vi "Simulation_Engine.vi"(0 "Path in":refnum<vi>, 1 "c_s2 [ppmv]":dbl=1.0, 2 "l2 [m]":dbl=1000.0, 3 "l_s [m]":dbl=0.1, 4 "c_s [ppmv]":dbl=1.0, 5 "c [ppmv]":dbl=1.7, 6 "l [m]":dbl=1000.0, 8 "c2 [ppmv]":dbl=7750.0, 9 "Array in":dbl[](array[numeric]), 10 "reference in":refnum<vi>, 11 "R":dbl, 12 "l_S2 [m]":dbl=1.0, 13 "K":dbl, 15 "Boolean":bool, 17 "f_LP1":dbl=1000.0, 19 "f_LP2":dbl=1000.0) -> (7 "I_OUT":cluster{dbl[], dbl[]}(graph), 14 "XY Graph":cluster{dbl[], dbl[]}[](graph), 16 "Widmo drugiej pochodnej":cluster{"f0":dbl, "df":dbl, "magnitude":dbl[]}(graph), 18 "Widmo pierwszej pochodnej":cluster{"f0":dbl, "df":dbl, "magnitude":dbl[]}(graph), 20 "Pierwsza pochodna":cluster{dbl[], dbl[]}(graph), 21 "Druga pochodna":cluster{dbl[], dbl[]}(graph), 23 "1fm":cluster{dbl[], dbl[]}(graph), 24 "2f bg":cluster{dbl[], dbl[]}(graph), 27 "2f/1f":cluster{dbl[], dbl[]}(graph))   [LabVIEW 2019]
uses:
  <vilib>/Analysis/3filter.llb/Filter Passband Type.ctl
  <vilib>/Utility/file.llb/Read Delimited Spreadsheet (DBL).vi
  <vilib>/Analysis/3filter.llb/Butterworth Filter (DBL).vi
  <vilib>/Analysis/baseanly.llb/IIR Cascade Filter (DBL).vi
  <vilib>/express/express analysis/Spectral/Block/exnSpectralBlock spectral measurements power poly.vi
  <vilib>/express/express analysis/Spectral/Block/exnSpectralBlock spectral measurements power WFM.vi
  <vilib>/express/express analysis/Spectral/XNode/ExpressSpectralMeasurementsBlockNode.xnode
  <vilib>/gmath/NI_Gmath.lvlib
  <vilib>/Analysis/NI_AALPro.lvlib
  <vilib>/Analysis/NI_AALBase.lvlib
panel:
  out "2f me":cluster{dbl[], dbl[]}(graph)
  out "1f bg":cluster{dbl[], dbl[]}(graph)
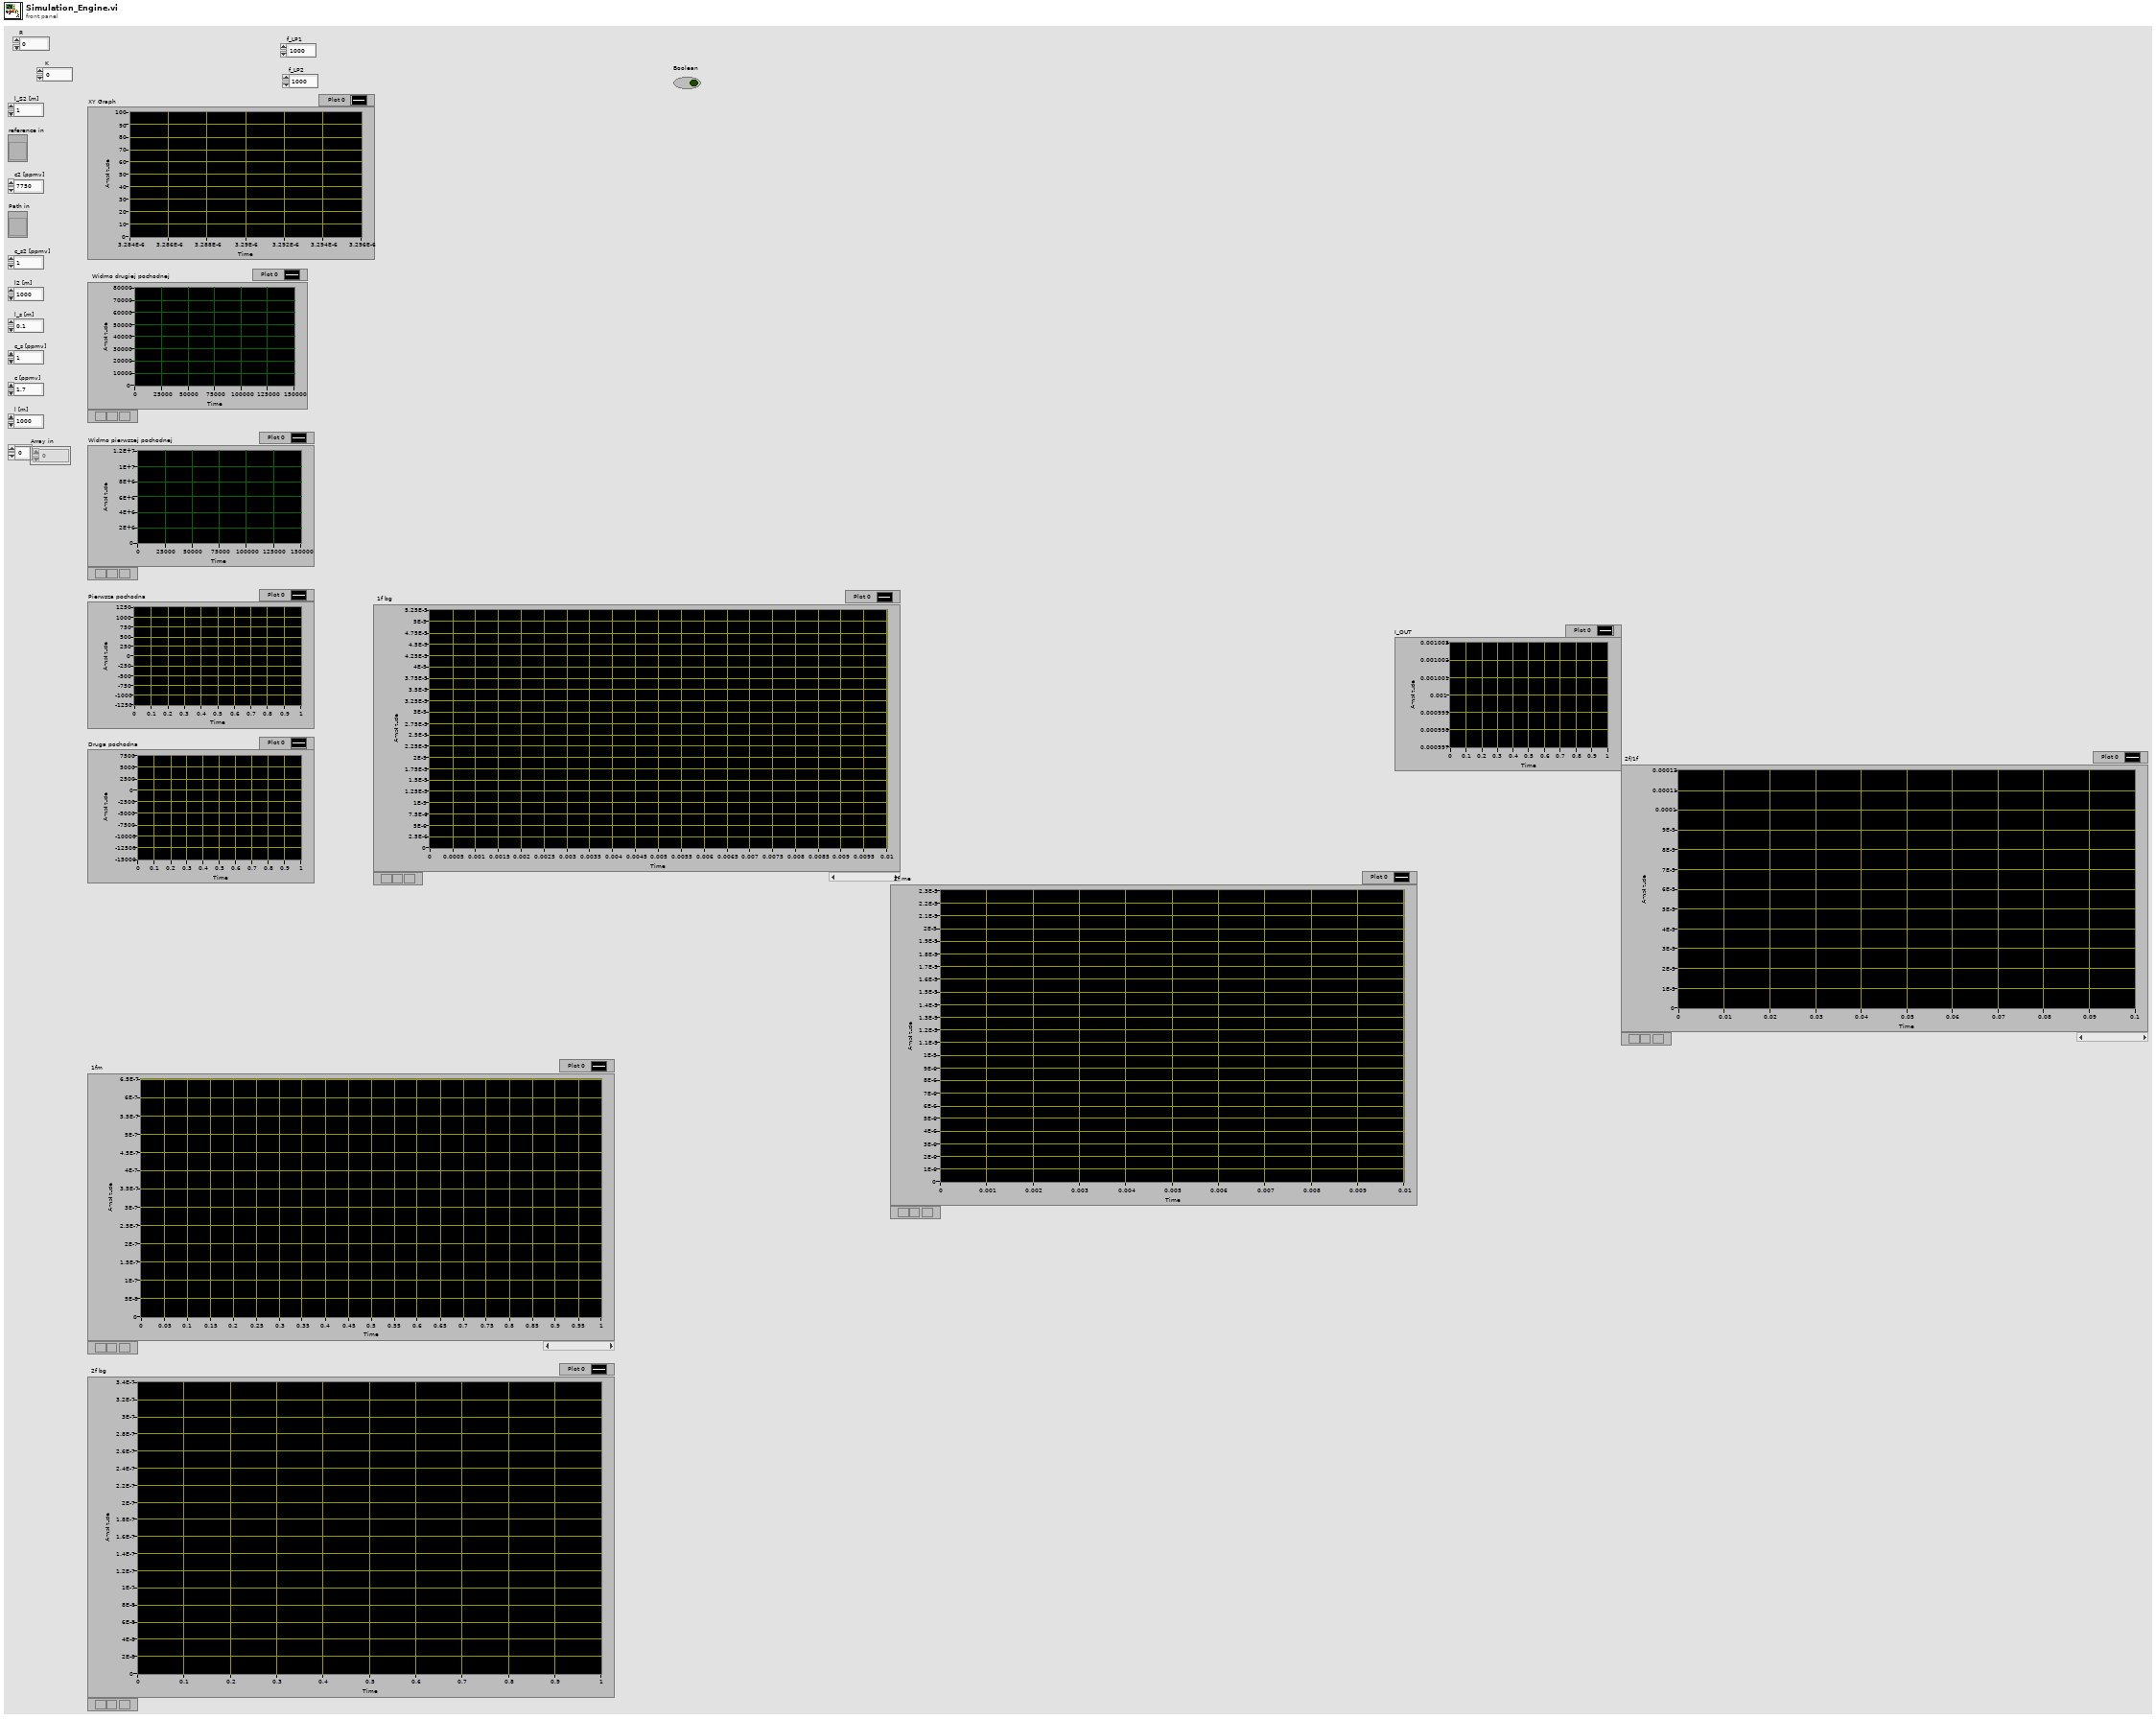
[diagram p1: front panel]
types:
  T1 = typedef "NI_AALBase.lvlib/Filter Passband Type.ctl" = enum32{"Lowpass", "Highpass", "Bandpass", "Bandstop"}
  T2 = cluster{"filter structure":enum32{"IIR 2nd Order", "IIR 4th Order"}, "Reverse Coefficients":dbl[], "Forward Coefficients":dbl[]}
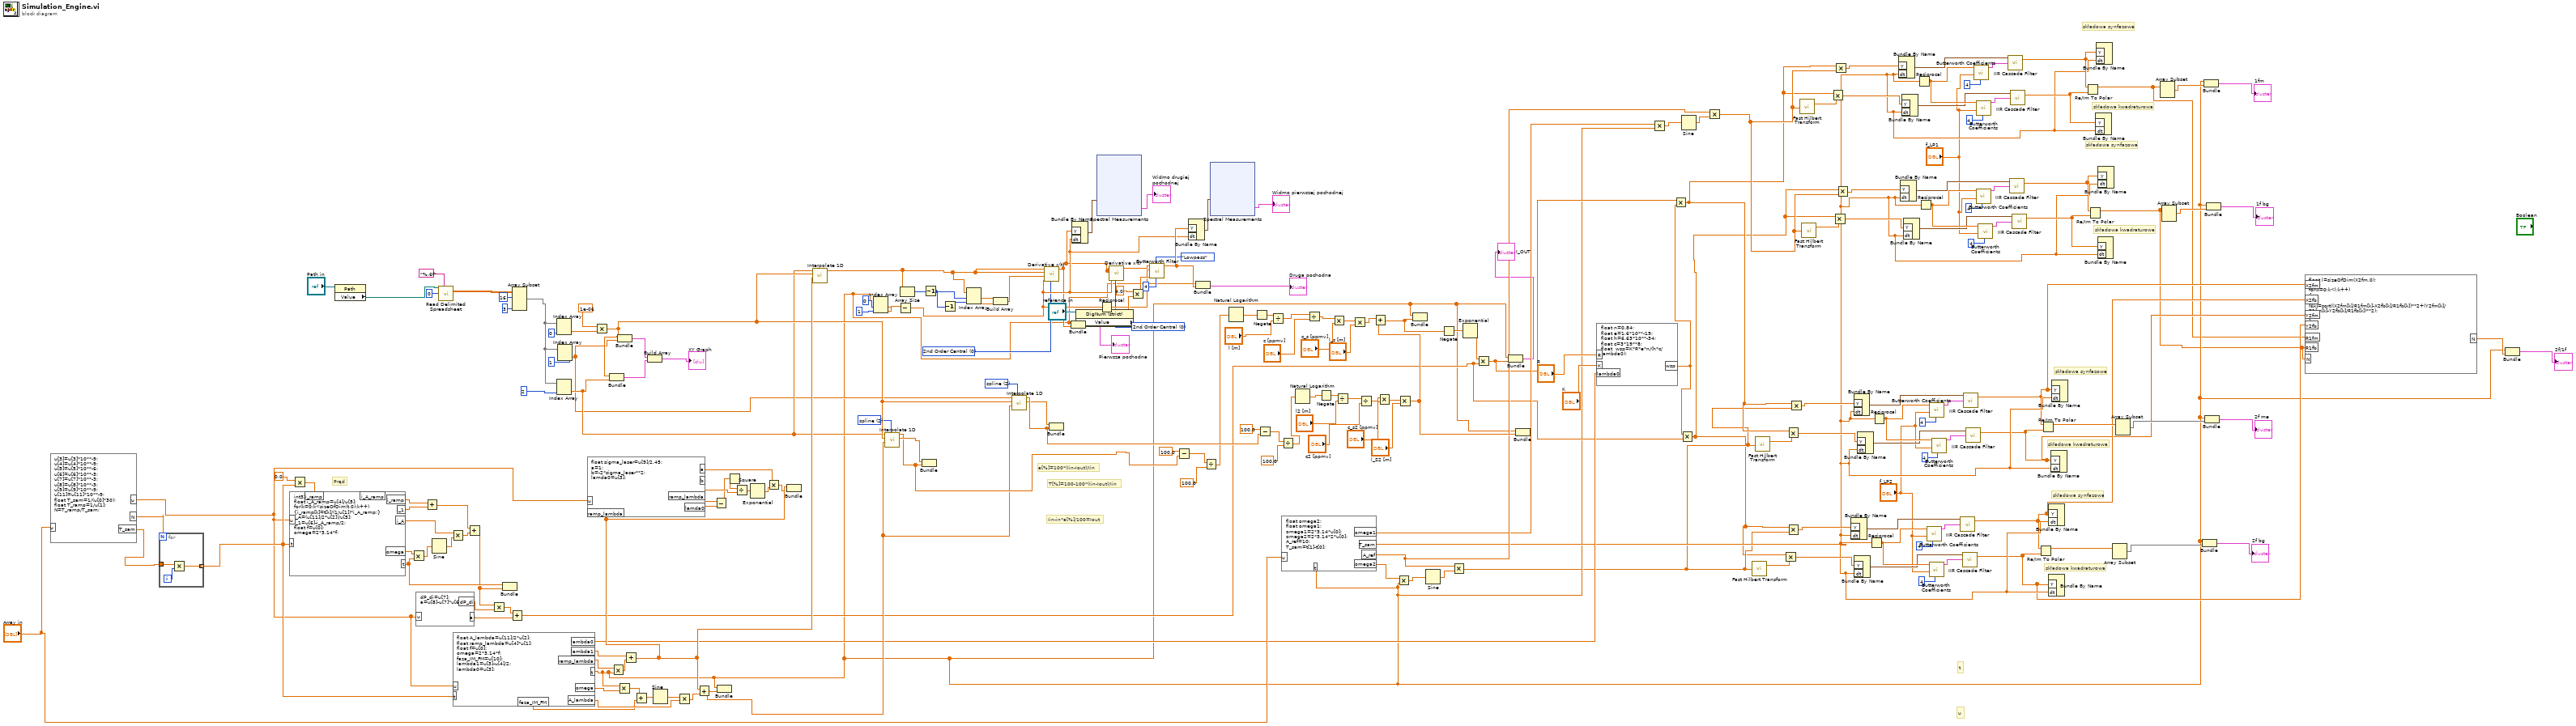
[diagram p0: block diagram]
diagram:
  w179 = u16 0 items=["2nd Order Central", "4th Order Central", "Forward", "Backward"] ("method")
  w170 = u16 0 items=["2nd Order Central", "4th Order Central", "Forward", "Backward"] ("method")
  w109 = 2 items=["nearest", "linear", "spline", "cubic Hermite", "Lagrange"] ("method")
  w106 = 2 items=["nearest", "linear", "spline", "cubic Hermite", "Lagrange"] ("method")
  # "składowa synfazowa"
  # "składowa synfazowa"
  # "składowa synfazowa"
  # "składowa kwadraturowa"
  # "składowa kwadraturowa"
  # "składowa kwadraturowa"
  # "składowa synfazowa"
  # "składowa kwadraturowa"
  # "u"
  # "t"
  # "T[%]=100-100*(Iin-Iout)/Iin"
  # "Iin-in*a[%]/100=Iout"
  # "a[%]=100*(Iin-Iout)/Iin"
  # "Natężenie"
  # "Prąd"
  n1 = formula code="u[3]=u[3]*10**-9;\nu[4]=u[4]*10**-9;\nu[5]=u[5]*10**-6;\nu[6]=u[6]*10**-3;\nu[7]=u[7]*10**-3;\nu[8]=u[8]*10**-3;\nu[9]=u[9]*10**-9;\nu[11]=u[11]*10**-9;\nfloat T_sam=1/(u[0]*30);\nfloat T_ramp=1/u[1];\nN=T_ramp/T_sam;"("u"="Array in") -> ("N"=w87:dbl, "T_sam"=w88:dbl, "u"=w89:dbl[])
  n2 = for {
    N: w87 -> [_]
    tunnel: w88 -> [w214]
    tunnel: [w212] -> w90 mode=indexing
    i -> [w213]
    n3 = Multiply(x=w214, y=w213) -> (x*y=w212:dbl)
  }
  n4 = Multiply(x=0.0, y=w90) -> (x*y=w56:dbl[])
  n5 = formula code="int32 k=0;\nfloat i_A_ramp=u[4]/u[5];\nfor(k=0;k<sizeOfDim(t,0);k++)\n{i_ramp[k]=t[k]/(1/u[1])*i_A_ramp;}\ni_A=(u[11]/2*u[2])/u[5];\ni_1=u[6]-i_A_ramp/2;\nfloat f=u[0];\nomega=2*3.14*f;"("u"=w89, "t"=w90, "i_ramp"=w56) -> ("i_A"=w57:dbl, "i_1"=w91:dbl, "i_ramp"=w59:dbl[], "omega"=w61:dbl, "t"=w190:dbl[])  [unwired: 1 out]
  n6 = property class="Path"(reference="Path in") -> ("Value"=w105:path)  [unwired: 1 in, 2 out]
  n7 = Multiply(x=w61, y=w190) -> (x*y=w62:dbl[])
  n8 = formula code="dP_di=u[7];\na=u[8]-u[7]*u[6];"("u"=w89) -> ("dP_di"=w65:dbl, "a"=w66:dbl)
  n9 = Add(x=w59, y=w91) -> (x+y=w60:dbl[])
  n10 = Sine(x=w62) -> (sin(x)=w63:dbl[])
  n11 = call-poly <vilib>:"Read Delimited Spreadsheet.vi"("file path (dialog if empty)"=w105, "format (%.3f)"="%.6f", "start of read offset (chars.:0)"=0) -> ("all rows"=w95:dbl[][])  [unwired: 7 in, 5 out]
  n12 = Multiply(x=w57, y=w63) -> (x*y=w58:dbl[])
  n13 = formula code="float A_lambda=u[11]/2*u[2];\nfloat ramp_lambda=u[4]*u[1];\nfloat f=u[0];\nomega=2*3.14*f;\nfaza_IM_FM=u[10];\nlambda1=u[3]-u[4]/2;\nlambda0=u[3];"("u"=w89, "t"=w90) -> ("ramp_lambda"=w74:dbl, "t"=w8:dbl[], "omega"=w68:dbl, "faza_IM_FM"=w70:dbl, "A_lambda"=w73:dbl, "lambda1"=w75:dbl, "lambda0"=w25:dbl)
  n14 = Add(x=w60, y=w58) -> (x+y=w64:dbl[])
  n15 = Multiply(x=w64, y=w65) -> (x*y=w67:dbl[])
  n16 = Bundle("t"=w190, w64) -> ()  [unwired: 1 in, 1 out]
  n17 = Add(x=w67, y=w66) -> (x+y=w21:dbl[])
  n18 = Array Subset(array=w95, index (row)=16 ("index"), length (col)=3 ("length")) -> (w94:dbl[][])  [unwired: 2 in]
  n19 = Index Array(array=w94, index (col)=2 ("disabled index (col)")) -> (element=w162:dbl[])  [unwired: 1 in]
  n20 = Index Array(array=w94, index (col)=0 ("disabled index (col)")) -> (element=w107:dbl[])  [unwired: 1 in]
  n21 = Index Array(array=w94, index (col)=1 ("disabled index (col)")) -> (element=w110:dbl[])  [unwired: 1 in]
  n22 = Multiply(x=1e-06, y=w107) -> (x*y=w163:dbl[])
  n23 = Bundle(w163, w162) -> (w93:cluster{dbl[], dbl[]})  [unwired: 1 in]
  n24 = Multiply(x=w74, y=w8) -> (x*y=w85:dbl[])
  n25 = Bundle(w163, w110) -> (w96:cluster{dbl[], dbl[]})  [unwired: 1 in]
  n26 = Multiply(x=w8, y=w68) -> (x*y=w69:dbl[])
  n27 = Add(x=w75, y=w85) -> (x+y=w169:dbl[])
  n28 = formula code="float sigma_laser=u[9]/2.45;\na=1;\nb=-2*sigma_laser**2;\nlamda0=u[3];"("u"=w89, "ramp_lambda"=w169) -> ("b"=w83:dbl, "a"=w78:dbl, "ramp_lambda"=w79:dbl[], "lamda0"=w80:dbl)
  n29 = Add(x=w69, y=w70) -> (x+y=w71:dbl[])
  n30 = Build Array(w96, w93) -> (→"XY Graph":cluster{dbl[], dbl[]}[])
  n31 = Sine(x=w71) -> (sin(x)=w72:dbl[])
  n32 = Multiply(x=w72, y=w73) -> (x*y=w76:dbl[])
  n33 = Add(x=w169, y=w76) -> (x+y=w111:dbl[])
  n34 = Subtract(x=w79, y=w80) -> (x-y=w81:dbl[])
  n35 = Bundle("t"=w8, w111) -> ()  [unwired: 1 in, 1 out]
  n36 = Square(x=w81) -> (x^2=w82:dbl[])
  n37 = Divide(x=w82, y=w83) -> (x/y=w84:dbl[])
  n38 = Exponential(1:w84) -> (0:w77:dbl[])
  n39 = Multiply(x=w78, y=w77) -> (x*y=w86:dbl[])
  n40 = Bundle(w169, w86) -> ()  [unwired: 1 in, 1 out]
  n41 = call <vilib>:"Interpolate 1D.vi"("xi"=w169, "X"=w163, "Y"=w162) -> ("yi"=w171:dbl[])  [unwired: 6 in, 2 out]
  n42 = Index Array(array=w8, index #1=0 ("index"), index #2=1 ("index")) -> (element #1=w164:dbl, element #2=w165:dbl)
  n43 = call <vilib>:"Interpolate 1D.vi"("method"=w106, "xi"=w111, "X"=w163, "Y"=w162) -> ("xi used"=w161:dbl[], "yi"=w160:dbl[])  [unwired: 5 in, 1 out]
  n44 = Subtract(x=w165, y=w164) -> (x-y=w191:dbl)
  n45 = Array Size(array=w171) -> (size(s)=w176:i32)
  n46 = Bundle("xi used"=w161, "yi"=w160) -> ()  [unwired: 1 in, 1 out]
  n47 = Decrement(x=w176) -> (x-1=w177:i32)
  n48 = Decrement(x=w177) -> (x-1=w172:i32)
  n49 = Index Array(array=w171, index #1=w177, index #2=w172) -> (element #1=w173:dbl, element #2=w174:dbl)
  n50 = Build Array(w173, w174) -> (w175:dbl[])
  n51 = call <vilib>:"Interpolate 1D.vi"("method"=w109, "xi"=w111, "X"=w163, "Y"=w110) -> ("xi used"=w108:dbl[], "yi"=w140:dbl[])  [unwired: 5 in, 1 out]
  n52 = call <vilib>:"Derivative x(t).vi"("method"=w170, "dt"=w191, "Final Condition"=w175, "Initial Condition"=w171, "X"=w171) -> ("dX/dt"=w186:dbl[])  [unwired: 5 in, 1 out]
  n53 = Bundle("xi used"=w108, "yi"=w140) -> ()  [unwired: 1 in, 1 out]
  n54 = Bundle("t"=w8, "dX/dt"=w186) -> (→"Pierwsza pochodna":cluster{"t":dbl[], "dX/dt":dbl[]})  [unwired: 1 in]
  n55 = Bundle By Name("Y"=w186, "dt"=w191) -> (w187:waveform(dbl))  [unwired: 1 in]
  n56 = property class="DigNum (strict)"(reference="reference in") -> ("Value"=w188:dbl)  [unwired: 1 in, 2 out]
  n57 = xnode "Spectral Measurements"("Signals"=w187) -> ("Power Spectrum"=→"Widmo drugiej pochodnej":cluster{"f0":dbl, "df":dbl, "magnitude":dbl[]})  [unwired: 1 in, 1 out]
  n58 = Reciprocal(x=w191) -> (1/x=w183:dbl)
  n59 = call <vilib>:"Derivative x(t).vi"("method"=w179, "dt"=w191, "Initial Condition"=w186, "X"=w186) -> ("dX/dt"=w180:dbl[])  [unwired: 6 in, 1 out]
  n60 = Multiply(x=4.0, y=w188) -> (x*y=w189:dbl)
  n61 = call-poly <vilib>:"Butterworth Filter.vi"("order"=4, "filter type"=Filter_Passband_Type."Lowpass", "low cutoff freq: fl"=w189, "sampling freq: fs"=w183, "X"=w180) -> ("Filtered X"=w192:dbl[])  [unwired: 3 in, 1 out]
  n62 = Subtract(x=100.0, y=w160) -> (x-y=w115:dbl[])
  n63 = Bundle By Name("Y"=w192, "dt"=w191) -> (w193:waveform(dbl))  [unwired: 1 in]
  n64 = Bundle("t"=w8, "Filtered X"=w192) -> (→"Druga pochodna":cluster{"t":dbl[], "Filtered X":dbl[]})  [unwired: 1 in]
  n65 = Divide(x=w115, y=100.0) -> (x/y=w116:dbl[])
  n66 = xnode "Spectral Measurements"("Signals"=w193) -> ("Power Spectrum"=→"Widmo pierwszej pochodnej":cluster{"f0":dbl, "df":dbl, "magnitude":dbl[]})  [unwired: 1 in, 1 out]
  n67 = Natural Logarithm(1:w116) -> (0:w113:dbl[])
  n68 = Negate(x=w113) -> (-x=w209:dbl[])
  n69 = Subtract(x=100.0, y=w140) -> (x-y=w138:dbl[])
  n70 = Divide(x=w209, y="l [m]") -> (x/y=w112:dbl[])
  n71 = Divide(x=w138, y=100.0) -> (x/y=w143:dbl[])
  n72 = formula code="float omega2;\nfloat omega1;\nomega1=2*3.14*u[0];\nomega2=2*3.14*2*u[0];\nA_ref=10;\nT_sam=t[1]-t[0];"("u"="Array in", "t"=w8) -> ("A_ref"=w159:dbl, "omega2"=w122:dbl, "T_sam"=w19:dbl, "omega1"=w26:dbl)
  n73 = Natural Logarithm(1:w143) -> (0:w142:dbl[])
  n74 = Divide(x=w112, y="c [ppmv]") -> (x/y=w199:dbl[])
  n75 = Negate(x=w142) -> (-x=w208:dbl[])
  n76 = Multiply(x=w199, y="c_s [ppmv]") -> (x*y=w200:dbl[])
  n77 = Divide(x=w208, y="l2 [m]") -> (x/y=w141:dbl[])
  n78 = Multiply(x=w200, y="l_s [m]") -> (x*y=w210:dbl[])
  n79 = Divide(x=w141, y="c2 [ppmv]") -> (x/y=w205:dbl[])
  n80 = Multiply(x=w205, y="c_s2 [ppmv]") -> (x*y=w203:dbl[])
  n81 = Multiply(x=w122, y=w8) -> (x*y=w134:dbl[])
  n82 = Multiply(x=w203, y="l_S2 [m]") -> (x*y=w204:dbl[])
  n83 = Add(x=w210, y=w204) -> (x+y=w144:dbl[])
  n84 = Bundle("t"=w8, w144) -> ()  [unwired: 1 in, 1 out]
  n85 = Sine(x=w134) -> (sin(x)=w135:dbl[])
  n86 = Negate(x=w144) -> (-x=w118:dbl[])
  n87 = Multiply(x=w159, y=w135) -> (x*y=w4:dbl[])
  n88 = Exponential(1:w118) -> (0:w119:dbl[])
  n89 = Multiply(x=w119, y=w21) -> (x*y=w22:dbl[])
  n90 = Bundle("t"=w8, w22) -> (→"I_OUT":cluster{"t":dbl[], dbl[]})  [unwired: 1 in]
  n91 = Bundle("t"=w8, w204) -> ()  [unwired: 1 in, 1 out]
  n92 = formula code="float n=0.84;\nfloat e=1.6*10**-19;\nfloat h=6.63*10**-34;\nfloat c=3*19**8;\nfloat  wsp=K*R*e*n/(h*c/lambda0);"("R"="R", "K"="K", "lambda0"=w25) -> ("wsp"=w20:dbl)
  n93 = Multiply(x=w26, y=w8) -> (x*y=w157:dbl[])
  n94 = Multiply(x=w22, y=w20) -> (x*y=w5:dbl[])
  n95 = Multiply(x=w20, y=w21) -> (x*y=w3:dbl[])
  n96 = Sine(x=w157) -> (sin(x)=w158:dbl[])
  n97 = Multiply(x=w159, y=w158) -> (x*y=w6:dbl[])
  n98 = call <vilib>:"Fast Hilbert Transform.vi"("X"=w4) -> ("Hilbert{X}"=w121:dbl[])  [unwired: 1 out]
  n99 = call <vilib>:"Fast Hilbert Transform.vi"("X"=w4) -> ("Hilbert{X}"=w27:dbl[])  [unwired: 1 out]
  n100 = Multiply(x=w3, y=w121) -> (x*y=w124:dbl[])
  n101 = Multiply(x=w5, y=w27) -> (x*y=w29:dbl[])
  n102 = Multiply(x=w3, y=w4) -> (x*y=w123:dbl[])
  n103 = Multiply(x=w5, y=w4) -> (x*y=w28:dbl[])
  n104 = call <vilib>:"Fast Hilbert Transform.vi"("X"=w6) -> ("Hilbert{X}"=w145:dbl[])  [unwired: 1 out]
  n105 = call <vilib>:"Fast Hilbert Transform.vi"("X"=w6) -> ("Hilbert{X}"=w40:dbl[])  [unwired: 1 out]
  n106 = Multiply(x=w5, y=w145) -> (x*y=w147:dbl[])
  n107 = Multiply(x=w3, y=w40) -> (x*y=w42:dbl[])
  n108 = Multiply(x=w5, y=w6) -> (x*y=w146:dbl[])
  n109 = Multiply(x=w3, y=w6) -> (x*y=w41:dbl[])
  n110 = Bundle By Name("Y"=w123, "dt"=w19) -> (w126:waveform(dbl))  [unwired: 1 in]
  n111 = Bundle By Name("Y"=w28, "dt"=w19) -> (w31:waveform(dbl))  [unwired: 1 in]
  n112 = Bundle By Name("Y"=w124, "dt"=w19) -> (w127:waveform(dbl))  [unwired: 1 in]
  n113 = Bundle By Name("Y"=w29, "dt"=w19) -> (w32:waveform(dbl))  [unwired: 1 in]
  n114 = Reciprocal(x=w19) -> (1/x=w131:dbl)
  n115 = Reciprocal(x=w19) -> (1/x=w36:dbl)
  n116 = Bundle By Name("Y"=w146, "dt"=w19) -> (w149:waveform(dbl))  [unwired: 1 in]
  n117 = Bundle By Name("Y"=w41, "dt"=w19) -> (w44:waveform(dbl))  [unwired: 1 in]
  n118 = Bundle By Name("Y"=w147, "dt"=w19) -> (w150:waveform(dbl))  [unwired: 1 in]
  n119 = Bundle By Name("Y"=w42, "dt"=w19) -> (w45:waveform(dbl))  [unwired: 1 in]
  n120 = Reciprocal(x=w19) -> (1/x=w154:dbl)
  n121 = Reciprocal(x=w19) -> (1/x=w49:dbl)
  n122 = call <vilib>:"Butterworth Coefficients.vi"("order"=4, "low cutoff freq: fl"="f_LP2", "sampling freq: fs"=w131) -> ("IIR Filter Cluster"=w125:T2)  [unwired: 7 in, 1 out]
  n123 = call <vilib>:"Butterworth Coefficients.vi"("order"=4, "low cutoff freq: fl"="f_LP2", "sampling freq: fs"=w131) -> ("IIR Filter Cluster"=w128:T2)  [unwired: 7 in, 1 out]
  n124 = call <vilib>:"Butterworth Coefficients.vi"("order"=4, "low cutoff freq: fl"="f_LP2", "sampling freq: fs"=w36) -> ("IIR Filter Cluster"=w30:T2)  [unwired: 7 in, 1 out]
  n125 = call <vilib>:"Butterworth Coefficients.vi"("order"=4, "low cutoff freq: fl"="f_LP2", "sampling freq: fs"=w36) -> ("IIR Filter Cluster"=w33:T2)  [unwired: 7 in, 1 out]
  n126 = call-poly <vilib>:"IIR Cascade Filter.vi"("IIR Filter Cluster"=w125, "X"=w126) -> ("Filtered X"=w15:dbl[])  [unwired: 1 in, 1 out]
  n127 = call-poly <vilib>:"IIR Cascade Filter.vi"("IIR Filter Cluster"=w128, "X"=w127) -> ("Filtered X"=w13:dbl[])  [unwired: 1 in, 1 out]
  n128 = call-poly <vilib>:"IIR Cascade Filter.vi"("IIR Filter Cluster"=w30, "X"=w31) -> ("Filtered X"=w16:dbl[])  [unwired: 1 in, 1 out]
  n129 = call-poly <vilib>:"IIR Cascade Filter.vi"("IIR Filter Cluster"=w33, "X"=w32) -> ("Filtered X"=w14:dbl[])  [unwired: 1 in, 1 out]
  n130 = call <vilib>:"Butterworth Coefficients.vi"("order"=4, "low cutoff freq: fl"="f_LP1", "sampling freq: fs"=w154) -> ("IIR Filter Cluster"=w148:T2)  [unwired: 7 in, 1 out]
  n131 = call <vilib>:"Butterworth Coefficients.vi"("order"=4, "low cutoff freq: fl"="f_LP1", "sampling freq: fs"=w49) -> ("IIR Filter Cluster"=w43:T2)  [unwired: 7 in, 1 out]
  n132 = call <vilib>:"Butterworth Coefficients.vi"("order"=4, "low cutoff freq: fl"="f_LP1", "sampling freq: fs"=w154) -> ("IIR Filter Cluster"=w151:T2)  [unwired: 7 in, 1 out]
  n133 = call <vilib>:"Butterworth Coefficients.vi"("order"=4, "low cutoff freq: fl"="f_LP1", "sampling freq: fs"=w49) -> ("IIR Filter Cluster"=w46:T2)  [unwired: 7 in, 1 out]
  n134 = call-poly <vilib>:"IIR Cascade Filter.vi"("IIR Filter Cluster"=w148, "X"=w149) -> ("Filtered X"=w155:dbl[])  [unwired: 1 in, 1 out]
  n135 = call-poly <vilib>:"IIR Cascade Filter.vi"("IIR Filter Cluster"=w43, "X"=w44) -> ("Filtered X"=w50:dbl[])  [unwired: 1 in, 1 out]
  n136 = call-poly <vilib>:"IIR Cascade Filter.vi"("IIR Filter Cluster"=w151, "X"=w150) -> ("Filtered X"=w156:dbl[])  [unwired: 1 in, 1 out]
  n137 = call-poly <vilib>:"IIR Cascade Filter.vi"("IIR Filter Cluster"=w46, "X"=w45) -> ("Filtered X"=w51:dbl[])  [unwired: 1 in, 1 out]
  n138 = Re/Im To Polar(2:w13, 3:w15) -> (1:w132:dbl[])  [unwired: 1 out]
  n139 = Re/Im To Polar(2:w14, 3:w16) -> (1:w37:dbl[])  [unwired: 1 out]
  n140 = Bundle By Name("Y"=w13, "dt"=w19) -> ()  [unwired: 1 in, 1 out]
  n141 = Bundle By Name("Y"=w15, "dt"=w19) -> ()  [unwired: 1 in, 1 out]
  n142 = Bundle By Name("Y"=w14, "dt"=w19) -> ()  [unwired: 1 in, 1 out]
  n143 = Bundle By Name("Y"=w16, "dt"=w19) -> ()  [unwired: 1 in, 1 out]
  n144 = Re/Im To Polar(2:w156, 3:w155) -> (1:w2:dbl[])  [unwired: 1 out]
  n145 = Re/Im To Polar(2:w51, 3:w50) -> (1:w1:dbl[])  [unwired: 1 out]
  n146 = Bundle By Name("Y"=w156, "dt"=w19) -> ()  [unwired: 1 in, 1 out]
  n147 = Bundle By Name("Y"=w155, "dt"=w19) -> ()  [unwired: 1 in, 1 out]
  n148 = Bundle By Name("Y"=w51, "dt"=w19) -> ()  [unwired: 1 in, 1 out]
  n149 = Bundle By Name("Y"=w50, "dt"=w19) -> ()  [unwired: 1 in, 1 out]
  n150 = Array Subset(array=w132) -> (w136:dbl[])  [unwired: 2 in]
  n151 = Array Subset(array=w37) -> (w39:dbl[])  [unwired: 2 in]
  n152 = Array Subset(array=w2) -> (w12:dbl[])  [unwired: 2 in]
  n153 = Array Subset(array=w1) -> (w11:dbl[])  [unwired: 2 in]
  n154 = Bundle("t"=w8, w136) -> (→"2f bg":cluster{"t":dbl[], dbl[]})  [unwired: 1 in]
  n155 = Bundle("t"=w8, w12) -> (→"1fm":cluster{"t":dbl[], dbl[]})  [unwired: 1 in]
  n156 = Bundle("t"=w8, w39) -> (→"2f me":cluster{"t":dbl[], dbl[]})  [unwired: 1 in]
  n157 = Bundle("t"=w8, w11) -> (→"1f bg":cluster{"t":dbl[], dbl[]})  [unwired: 1 in]
  n158 = formula code="float l=sizeOfDim(X2fm,0);\nint k;\nfor(k=0;k<l;k++)\n{\n\nN[k]=sqrt((X2fm[k]/R1fm[k]-X2fb[k]/R1fb[k])**2+(Y2fm[k]/R1fm[k]-Y2fb[k]/R1fb[k])**2);\n\n}"("X2fm"=w16, "X2fb"=w15, "Y2fm"=w14, "Y2fb"=w13, "R1fm"=w2, "R1fb"=w1, "N"=w1) -> ("N"=w9:dbl[])
  n159 = Bundle("t"=w8, "N"=w9) -> (→"2f/1f":cluster{"t":dbl[], "N":dbl[]})  [unwired: 1 in]
